vi "Configure Regulation Gain.vi"(0 "VISA resource name":refnum<visa-resource-name>, 5 "Regulation Gain (0)":dbl format="%#.6f", 11 "error in (no error)":errorcluster) -> (4 "VISA resource name out":refnum<visa-resource-name>, 15 "error out":errorcluster)   [LabVIEW 2020, in "NH Research Regenerative Test Series.lvlib"]
doc: "Sets the percent correction applied during each control loop to regulate the output. A value of 0 will inhibit the regulation feedback. The larger the value the bigger the adjustment. The value is a percent entered as a floating point where 5% is 0.05."
uses:
  NH Research Regenerative Test Series.lvlib
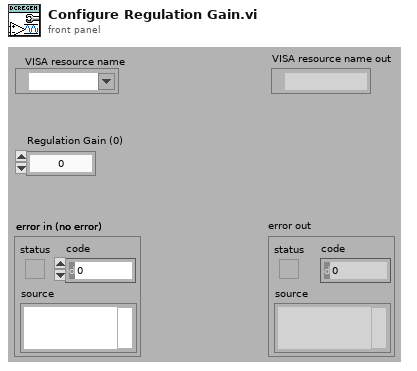
[diagram p1: front panel]
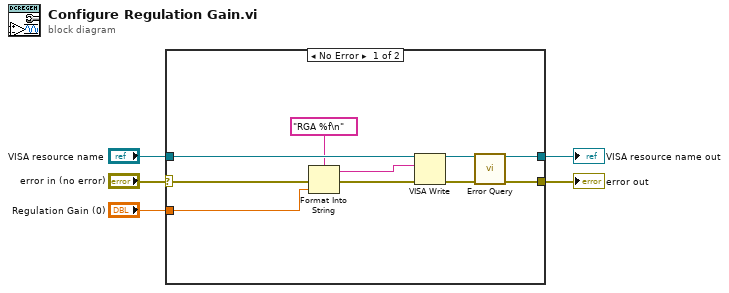
[diagram p0: block diagram]
diagram:
  n1 = case shown="No Error" "error in (no error)" {
    selector: "error in (no error)" -> [w10 w17]
    tunnel: "VISA resource name" -> [w15 w16]
    tunnel: [w12 w16] -> w4
    tunnel: [w11 w17] -> w3
    tunnel: "Regulation Gain (0)" -> [w6 _]
    frame No Error {
      n2 = Format Into String(format string="RGA %f\n" ("Command"), error in=w10, w6) -> (resulting string=w13:string, error out=w9:errorcluster)  [unwired: 1 in]
      n3 = VISA Write(VISA resource name=w15, write buffer=w13, error in (no error)=w9) -> (VISA resource name out=w8:refnum<visa-resource-name>, error out=w7:errorcluster)  [unwired: 1 out]
      n4 = call "Error Query.vi"("VISA resource name"=w8, "error in (no error)"=w7) -> ("VISA resource name out"=w12:refnum<visa-resource-name>, "error out"=w11:errorcluster)  [unwired: 10 in, 2 out]
    }
    frame Error {
    }
  }
  "error out" <- w3
  "VISA resource name out" <- w4
